vi "Init.vi"(8 "error in (no error)":errorcluster, 10 "Topic":string, 11 "Pub Sub Event Channel in":refnum<class "Pub Sub Event Channel.lvclass">) -> (0 "error out":errorcluster, 3 "Pub Sub Event Channel out":refnum<class "Pub Sub Event Channel.lvclass">)   [LabVIEW 2020, in "Actor Pub Sub Channels.lvlib" / "Pub Sub Event Channel.lvclass"]
uses:
  Pub Sub Event Channel.lvclass
  Pub Sub Event Channel.lvclass/Pub Sub Event Channel.ctl
  <vilib>/ActorFramework/Message/Message.lvclass
  Pub Sub Message Channel/Pub Sub Message Channel.lvclass
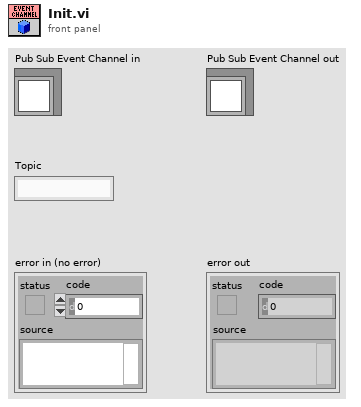
[diagram p1: front panel]
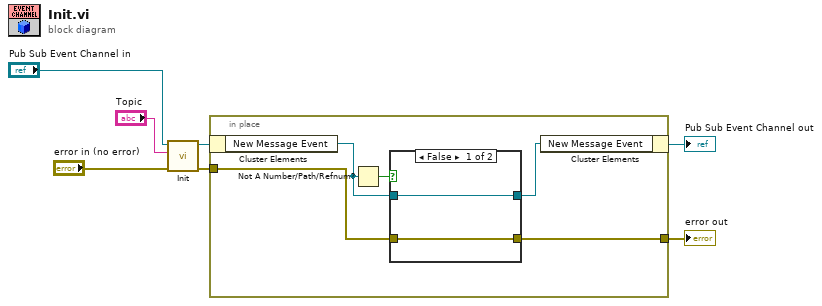
[diagram p0: block diagram]
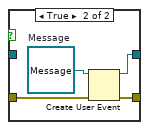
[diagram p2: hidden frame]
diagram:
  n1 = call-parent "Init.vi"("error in (no error)"="error in (no error)", "Topic"="Topic", "Pub Sub Message Channel in"="Pub Sub Event Channel in") -> ("error out"=w2:errorcluster, "Pub Sub Message Channel out"=w7:refnum<class "Pub Sub Event Channel.lvclass">)  [unwired: 7 in]
  n2 = in-place {
    in-place-border: w2 -> [w12]
    in-place-border: [w11] -> w1
    n3 = in-place-cluster #1(w7) -> ("New Message Event"=w8:refnum<user-event>)
    n4 = Not A Number/Path/Refnum?(number/path/refnum=w8) -> (NaN/Path/Refnum?=w10:bool)
    n5 = case shown="False" w10 {
      tunnel: w12 -> [w14 w18]
      tunnel: [w14 w17] -> w11
      tunnel: [w13 w15] -> w9
      tunnel: w8 -> [w13 _]
      frame False {
      }
      frame True {
        w16 = refnum<class "Message.lvclass"> refnum  # Message
        n6 = Create User Event(user event datatype=w16, error in=w18) -> (user event=w15:refnum<user-event>, error out=w17:errorcluster)
      }
    }
    n7 = in-place-cluster #1("New Message Event"=w9) -> (→"Pub Sub Event Channel out":refnum<class "Pub Sub Event Channel.lvclass">)
  }
  "error out" <- w1
